vi "Save Parser Settings.vi"(8 "Error in":errorcluster caption="Error in (no error)", 10 "Parser Settings":T1 caption="Doc Options", 11 "Settings Path":path) -> (0 "Error out":errorcluster)   [LabVIEW 2023, in "VIDoc Parsing.lvlib" / "Parser Settings.lvclass"]
uses:
  Parser Settings.lvclass
  Parser Settings Cluster.ctl
  Draw Controls Cluster.ctl
  Draw Option Enum.ctl
  e450ed71-4968-4477-8672-58ac8a0708d9.vi
  <vilib>/JDP Science/JSONtext/Variant to JSON Text.vi
  <vilib>/JDP Science/JSONtext/LVClass Serializer/JSONtext LVClass Serializer.lvclass
  VIDoc Settings/VIDoc Settings.lvclass
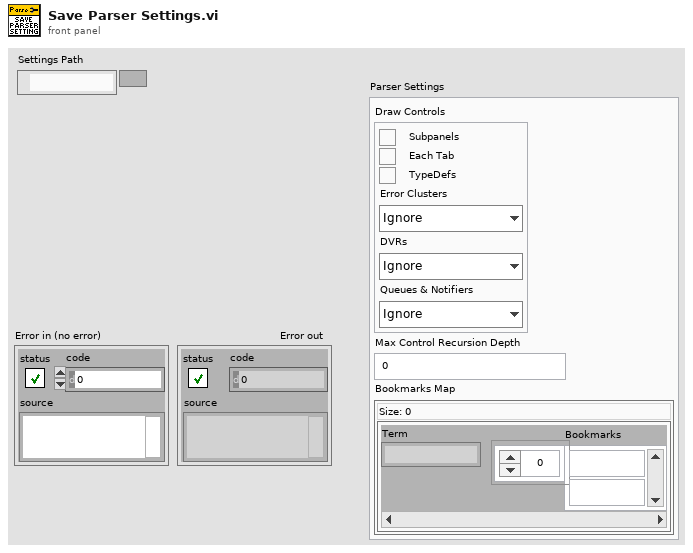
[diagram p1: front panel]
types:
  T1 = typedef "VIDoc Parsing.lvlib/Parser Settings.lvclass/Parser Settings Cluster.ctl" = cluster{"Draw Controls":T2, "Max Control Recursion Depth":i32, "Bookmarks Map":map{string, string[]}}
  T2 = typedef "VIDoc Parsing.lvlib/Parser Settings.lvclass/Draw Controls Cluster.ctl" = cluster{"Subpanels":bool, "Tabs":bool, "TypeDefs":bool, "Error Clusters":T3, "DVRs":T3, "Queues & Notifiers":T3}
  T3 = typedef "VIDoc Parsing.lvlib/Parser Settings.lvclass/Draw Option Enum.ctl" = enum16{"Ignore", "Draw", "Draw + Contents"}
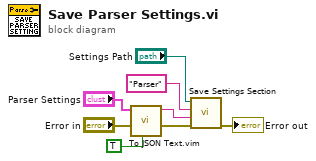
[diagram p0: block diagram]
diagram:
  n1 = call "To JSON Text.vim"("Pretty Print?"=TRUE, "error in (no error)"="Error in", "Anything"="Parser Settings") -> ("error out"=w6:errorcluster, "<JSON>"=w4:string)  [unwired: 7 in]
  n2 = call "Save Settings Section.vi"("Error in"=w6, "JSON Object"=w4, "Section Name"="Parser", "JSON Settings Path"="Settings Path") -> ("Error out"=→"Error out":errorcluster)  [unwired: 7 in]
